vi "RT_Thrust_Force_in_DLR_Navigation_Reference_System(SubVI).vi"(8 "Rotation":T1, 10 "FE_b":dbl[](array[numeric])) -> (3 "FE":dbl[](array[numeric]))   [LabVIEW 2017]
uses:
  <vilib>/Analysis/baseanly.llb/Real A x B.vi
  <vilib>/Analysis/Matrix/Numeric/Conversions/Array To Matrix - RA.vi
  <vilib>/Analysis/Matrix/Numeric/Conversions/Array To Matrix - RA2.vi
  <vilib>/Analysis/Matrix/Numeric/Conversions/Matrix To Array - RM.vi
  <vilib>/Analysis/Matrix/NI_Matrix.lvlib
  <vilib>/Analysis/NI_AALBase.lvlib
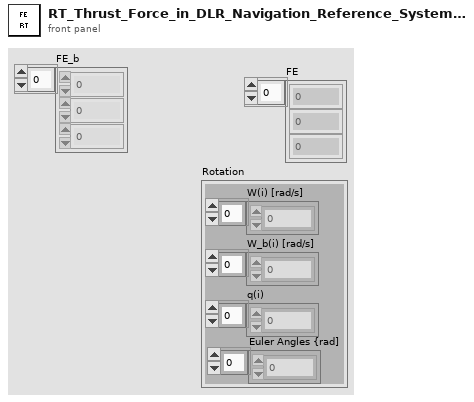
[diagram p1: front panel]
types:
  T1 = cluster{"W(i) [rad/s]":dbl[], "W_b(i) [rad/s]":dbl[], "q(i)":dbl[], "Euler Angles {rad]":dbl[]}
  T2 = typedef "NI_Matrix.lvlib/RealMatrix.ctl" = dbl[][]
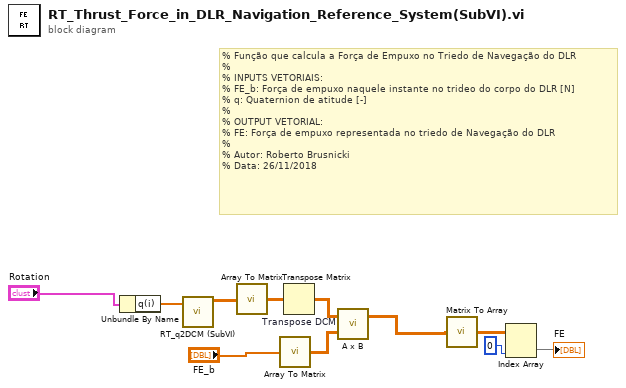
[diagram p0: block diagram]
diagram:
  # "% Função que calcula a Força de Empuxo no Triedo de Navegação do DLR \n%\n% INPUTS VETORIAIS:\n% FE_b: Força de empuxo naquele instante no trideo do corpo do DLR [N]\n% q: Quaternion de atitude\t[-]\n%\n% OUTPUT VETORIAL:\n% FE: Força de empuxo representada no triedo de Navegação do DLR\n%\n% Autor: Roberto Brusnicki\n% Data: 26/11/2018"
  n1 = Unbundle By Name("Rotation") -> ("q(i)"=w3:dbl[])
  n2 = call "RT_q2DCM (SubVI).vi"("Quaternion"=w3) -> ("DCM"=w2:dbl[][])  [unwired: 10 in]
  n3 = call-poly <vilib>:"Array To Matrix.vi"("Real 2D Array"=w2) -> ("Real Matrix"=w6:T2)
  n4 = call-poly <vilib>:"Array To Matrix.vi"("Real 1D Array"="FE_b") -> ("Real Matrix (Column Vector)"=w8:T2)
  n5 = Transpose Matrix "Transpose DCM"(1:w6) -> (0:w7:T2)
  n6 = call-poly <vilib>:"A x B.vi"("B"=w8, "A"=w7) -> ("A x B"=w5:T2)  [unwired: 1 out]
  n7 = call-poly <vilib>:"Matrix To Array.vi"("Real Matrix"=w5) -> ("Real 2D Array"=w11:dbl[][])
  n8 = Index Array(array=w11, index (col)=0 ("index (row)")) -> (element=→"FE":dbl[])  [unwired: 1 in]
